vi "Codec_CMD_WILL.vi"(8 "error in (no error)":errorcluster, 11 "SecureMqttCodec in":refnum<class "SecureMqttCodec.lvclass">) -> (0 "error out":errorcluster, 2 "<JSON>":string, 3 "SecureMqttCodec out":refnum<class "SecureMqttCodec.lvclass">)   [LabVIEW 2020, in "SecureMqttCodec.lvclass"]
uses:
  SecureMqttCodec.lvclass
  SecureMqttCodec.lvclass/SecureMqttCodec.ctl
  <vilib>/addons/JSON API/JSON Value/Set from JSON string.vi
  <vilib>/LabVIEW Open Source Project/Epoch Date & Time/epoch.UNIX/Epoch.UNIX.lvclass
  C:/Program Files/National Instruments/LabVIEW 2020/vi.lib/LabVIEW Open Source Project/Epoch Date & Time/epoch/Epoch.lvclass
  <vilib>/addons/JSON API/JSON Scalar/JSON Scalar.lvclass
  C:/Program Files/National Instruments/LabVIEW 2020/vi.lib/addons/JSON API/JSON Value/JSON Value.lvclass
  <vilib>/addons/JSON API/JSON Array/JSON Array.lvclass
  <vilib>/LabVIEW Open Source Project/Epoch Date & Time/Get Epoch Time.vi
  <vilib>/addons/JSON API/JSON Scalar/Set I64.vi
  <vilib>/addons/JSON API/JSON Scalar/Set U32.vi
  <vilib>/addons/JSON API/JSON Scalar/Set String.vi
  <vilib>/addons/JSON API/JSON Array/Set JSON Array.vi
  <vilib>/addons/JSON API/JSON Value/Get as JSON string (pretty).vi
  <vilib>/addons/JSON API/JSON Value/JSON Value.lvclass
  <vilib>/addons/JSON API/Get Polymorphic/JSON GetSet.lvlib
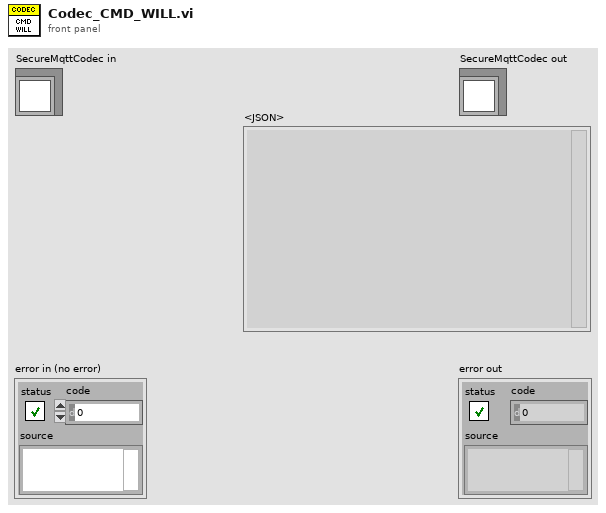
[diagram p1: front panel]
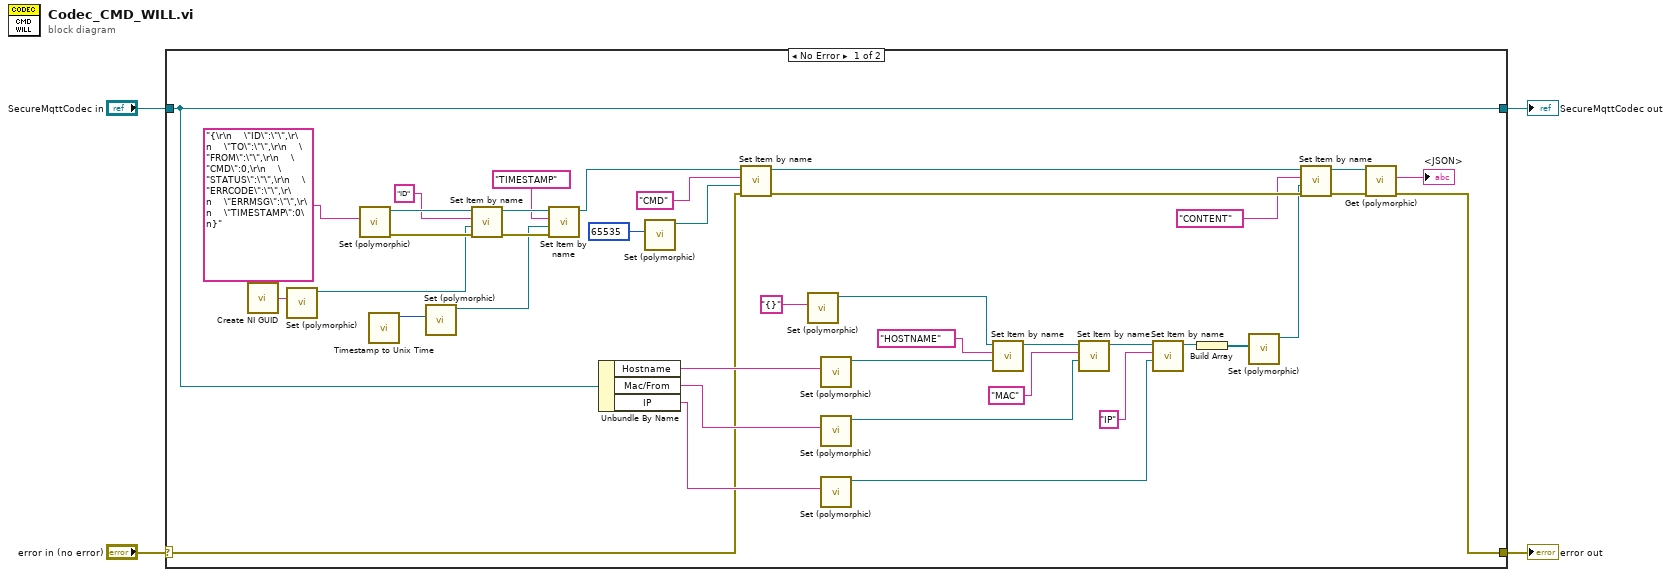
[diagram p0: block diagram]
diagram:
  n1 = case shown="No Error" "error in (no error)" {
    selector: "error in (no error)" -> [w18 w46]
    tunnel: [w41 w46] -> w3
    tunnel: [w44 w45] -> w1
    tunnel: "SecureMqttCodec in" -> [w44 w45]
    frame No Error {
      n2 = call <vilib>:"Create NI GUID.vi"() -> ("NI GUID"=w9:string)
      n3 = call-poly <vilib>:"Set (polymorphic).vi"("String"=w9) -> ("JSON Scalar out"=w10:refnum<class "JSON Scalar.lvclass">)  [unwired: 9 in, 1 out]
      n4 = call-poly <vilib>:"Set (polymorphic).vi"("JSON stream"="{\r\n    \"ID\":\"\",\r\n    \"TO\":\"\",\r\n    \"FROM\":\"\",\r\n    \"CMD\":0,\r\n    \"STATUS\":\"\",\r\n    \"ERRCODE\":\"\",\r\n    \"ERRMSG\":\"\",\r\n    \"TIMESTAMP\":0\n}" ("JSON String")) -> ("error out"=w12:errorcluster, "JSON Value out"=w11:refnum<class "JSON Value.lvclass">)  [unwired: 8 in, 1 out]
      n5 = call <vilib>:"Timestamp to Unix Time.vi"() -> ("Unix Time (s)"=w13:i64)  [unwired: 10 in, 1 out]
      n6 = call-poly <vilib>:"Set (polymorphic).vi"("Numeric"=w13) -> ("JSON Scalar out"=w14:refnum<class "JSON Scalar.lvclass">)  [unwired: 9 in, 1 out]
      n7 = call-dynamic "Set Item by name.vi"("error in (no error)"=w12, "Value"=w10, "name"="ID", "JSON Value In"=w11) -> ("error out"=w16:errorcluster, "JSON Value Out"=w15:refnum<class "JSON Value.lvclass">)  [unwired: 5 in, 1 out]
      n8 = call-dynamic "Set Item by name.vi"("error in (no error)"=w16, "Value"=w14, "name"="TIMESTAMP", "JSON Value In"=w15) -> ("JSON Value Out"=w5:refnum<class "JSON Value.lvclass">)  [unwired: 5 in, 2 out]
      n9 = Unbundle By Name(w44) -> ("Hostname"=w27:string, "Mac/From"=w26:string, "IP"=w25:string)
      n10 = call-poly <vilib>:"Set (polymorphic).vi"("Numeric"=u32 65535) -> ("JSON Scalar out"=w42:refnum<class "JSON Scalar.lvclass">)  [unwired: 9 in, 1 out]
      n11 = call-dynamic "Set Item by name.vi"("error in (no error)"=w18, "Value"=w42, "name"="CMD", "JSON Value In"=w5) -> ("error out"=w22:errorcluster, "JSON Value Out"=w24:refnum<class "JSON Value.lvclass">)  [unwired: 5 in, 1 out]
      n12 = call-poly <vilib>:"Set (polymorphic).vi"("JSON stream"="{}" ("JSON")) -> ("JSON Value out"=w39:refnum<class "JSON Value.lvclass">)  [unwired: 8 in, 2 out]
      n13 = call-poly <vilib>:"Set (polymorphic).vi"("String"=w27) -> ("JSON Scalar out"=w38:refnum<class "JSON Scalar.lvclass">)  [unwired: 9 in, 1 out]
      n14 = call-poly <vilib>:"Set (polymorphic).vi"("String"=w26) -> ("JSON Scalar out"=w35:refnum<class "JSON Scalar.lvclass">)  [unwired: 9 in, 1 out]
      n15 = call-poly <vilib>:"Set (polymorphic).vi"("String"=w25) -> ("JSON Scalar out"=w34:refnum<class "JSON Scalar.lvclass">)  [unwired: 9 in, 1 out]
      n16 = call-dynamic "Set Item by name.vi"("Value"=w38, "name"="HOSTNAME", "JSON Value In"=w39) -> ("JSON Value Out"=w37:refnum<class "JSON Value.lvclass">)  [unwired: 6 in, 2 out]
      n17 = call-dynamic "Set Item by name.vi"("Value"=w35, "name"="MAC", "JSON Value In"=w37) -> ("JSON Value Out"=w36:refnum<class "JSON Value.lvclass">)  [unwired: 6 in, 2 out]
      n18 = call-dynamic "Set Item by name.vi"("Value"=w34, "name"="IP", "JSON Value In"=w36) -> ("JSON Value Out"=w33:refnum<class "JSON Value.lvclass">)  [unwired: 6 in, 2 out]
      n19 = Build Array(w33) -> (w32:refnum<class "JSON Value.lvclass">[])
      n20 = call-poly <vilib>:"Set (polymorphic).vi"("Array"=w32) -> ("JSON Array out"=w20:refnum<class "JSON Array.lvclass">)  [unwired: 9 in, 1 out]
      n21 = call-dynamic "Set Item by name.vi"("error in (no error)"=w22, "Value"=w20, "name"="CONTENT", "JSON Value In"=w24) -> ("error out"=w21:errorcluster, "JSON Value Out"=w23:refnum<class "JSON Value.lvclass">)  [unwired: 5 in, 1 out]
      n22 = call-poly <vilib>:"Get (polymorphic).vi"("error in (no error)"=w21, "JSON Value in"=w23) -> ("error out"=w41:errorcluster, "<JSON>"=→"<JSON>":string)  [unwired: 8 in]
    }
    frame Error {
    }
  }
  "error out" <- w3
  "SecureMqttCodec out" <- w1
